vi "Slice 1D Array__ogtk.vi"   [LabVIEW 2018]
doc: "Returns a subset from <B>array</B>. <B>subset</B> has the following syntax:\n\narray[subset] = subarray\n\nsubset is a range and is of the form \"i:j\" where i and j are integers\nif i is ommitted it is assumed to be zero. If j is ommitted it is assumed to be length(array)\nif i or j are negative numbers they are assumed to be refferenced from the end of the string.\nexamples:\n\nif array = [7,6,5,4,3,2,1]\n\nstring[2:] = [5,4,3,2,1]\nstring[:3] = [7,6,5]\nstring[-1] = [1]\nstring[4] = [3]\nstring[-4:-2] = [4,3]"
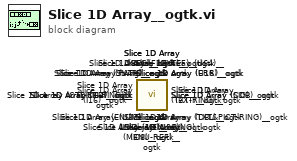
[diagram p0: block diagram]
diagram:
  n1 = call <userlib>:"Slice 1D Array (LVObject)__ogtk.vi"() -> ()  [unwired: 7 in, 1 out]
  n2 = call <userlib>:"Slice 1D Array (U64)__ogtk.vi"() -> ()  [unwired: 7 in, 1 out]
  n3 = call <userlib>:"Slice 1D Array (I64)__ogtk.vi"() -> ()  [unwired: 7 in, 1 out]
  n4 = call <userlib>:"Slice 1D Array (SIG)__ogtk.vi"() -> ()  [unwired: 7 in, 1 out]
  n5 = call <userlib>:"Slice 1D Array (String)__ogtk.vi"() -> ()  [unwired: 7 in, 1 out]
  n6 = call <userlib>:"Slice 1D Array (CSG)__ogtk.vi"() -> ()  [unwired: 7 in, 1 out]
  n7 = call <userlib>:"Slice 1D Array (DBL)__ogtk.vi"() -> ()  [unwired: 7 in, 1 out]
  n8 = call <userlib>:"Slice 1D Array (I16)__ogtk.vi"() -> ()  [unwired: 7 in, 1 out]
  n9 = call <userlib>:"Slice 1D Array (EXT)__ogtk.vi"() -> ()  [unwired: 7 in, 1 out]
  n10 = call <userlib>:"Slice 1D Array (I08)__ogtk.vi"() -> ()  [unwired: 7 in, 1 out]
  n11 = call <userlib>:"Slice 1D Array (U32)__ogtk.vi"() -> ()  [unwired: 7 in, 1 out]
  n12 = call <userlib>:"Slice 1D Array (U16)__ogtk.vi"() -> ()  [unwired: 7 in, 1 out]
  n13 = call <userlib>:"Slice 1D Array (U08)__ogtk.vi"() -> ()  [unwired: 7 in, 1 out]
  n14 = call <userlib>:"Slice 1D Array (CXT)__ogtk.vi"() -> ()  [unwired: 7 in, 1 out]
  n15 = call <userlib>:"Slice 1D Array (I32)__ogtk.vi"() -> ()  [unwired: 7 in, 1 out]
  n16 = call <userlib>:"Slice 1D Array (CDB)__ogtk.vi"() -> ()  [unwired: 7 in, 1 out]
  n17 = call <userlib>:"Slice 1D Array (PATH)__ogtk.vi"() -> ()  [unwired: 7 in, 1 out]
  n18 = call <userlib>:"Slice 1D Array (TXT&PICT-RING)__ogtk.vi"() -> ()  [unwired: 7 in, 1 out]
  n19 = call <userlib>:"Slice 1D Array (BOL)__ogtk.vi"() -> ()  [unwired: 7 in, 1 out]
  n20 = call <userlib>:"Slice 1D Array (ENUM)__ogtk.vi"() -> ()  [unwired: 7 in, 1 out]
  n21 = call <userlib>:"Slice 1D Array (MENU-RING)__ogtk.vi"() -> ()  [unwired: 7 in, 1 out]
  n22 = call <userlib>:"Slice 1D Array (PICT-RING)__ogtk.vi"() -> ()  [unwired: 7 in, 1 out]
  n23 = call <userlib>:"Slice 1D Array (TXT-RING)__ogtk.vi"() -> ()  [unwired: 7 in, 1 out]
  n24 = call <userlib>:"Slice 1D Array (ERR)__ogtk.vi"() -> ()  [unwired: 7 in, 1 out]
  n25 = call <userlib>:"Slice 1D Array (MENU-REF)__ogtk.vi"() -> ()  [unwired: 7 in, 1 out]
  n26 = call <userlib>:"Slice 1D Array (FILE-REF)__ogtk.vi"() -> ()  [unwired: 7 in, 1 out]
  n27 = call <userlib>:"Slice 1D Array (CTL-REF)__ogtk.vi"() -> ()  [unwired: 7 in, 1 out]
  n28 = call <userlib>:"Slice 1D Array (VAR)__ogtk.vi"() -> ()  [unwired: 7 in, 1 out]
